vi "CLEARPATH CONTROL SYSTEM 1 AXIS.vi"() -> ()   [LabVIEW 2014]
uses:
  Control 1.ctl
  54e35cf9-3849-4311-9828-ef4f6905ae2a.vi
  83293444-dc6f-4323-ab08-cbfa26563ffd.vi
  <vilib>/Instr/_visa.llb/VISA Flush IO Buffer Mask.ctl
  b9a6dcee-82f6-4e18-8d36-9c0f5dd18835.vi
  <vilib>/Instr/_visa.llb/VISA Configure Serial Port (Instr).vi
panel:
  in  "?":bool
  in  "Y Positions (0<Y<35)":dbl[](array[numeric])
  in  "X Positions (0<X<38)":dbl[](array[numeric])
  # "End Command:\n10000"
  # "There can be no values after 10000, causes the motor to rotate infinitely. To delete a cell, \nright click on the cell, then select, Data Operations -> Delete Element. \n10000 MUST BE THE LAST COMMAND."
  # "System operates by moving to a given Y-Value,\nthen iterates through all X values. After all Y-Values\nare complete the program waits for user confirmation\nthen returns to (0,0)."
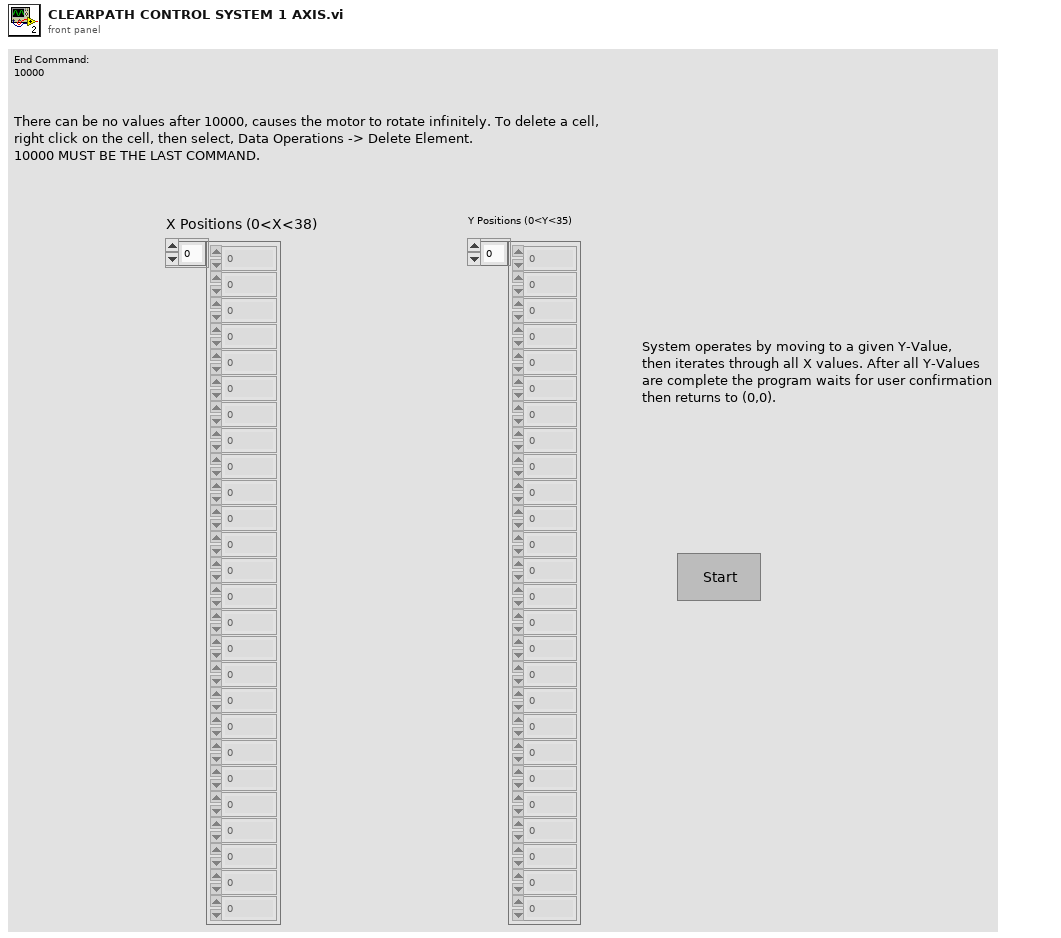
[diagram p1: front panel]
types:
  T1 = typedef "Control 1.ctl" = enum16{"Start", "Init", "Await Arduino Response", "Calculate Move", "Execute Move", "Home"}
  T2 = typedef "VISA Flush IO Buffer Mask.ctl" = u16
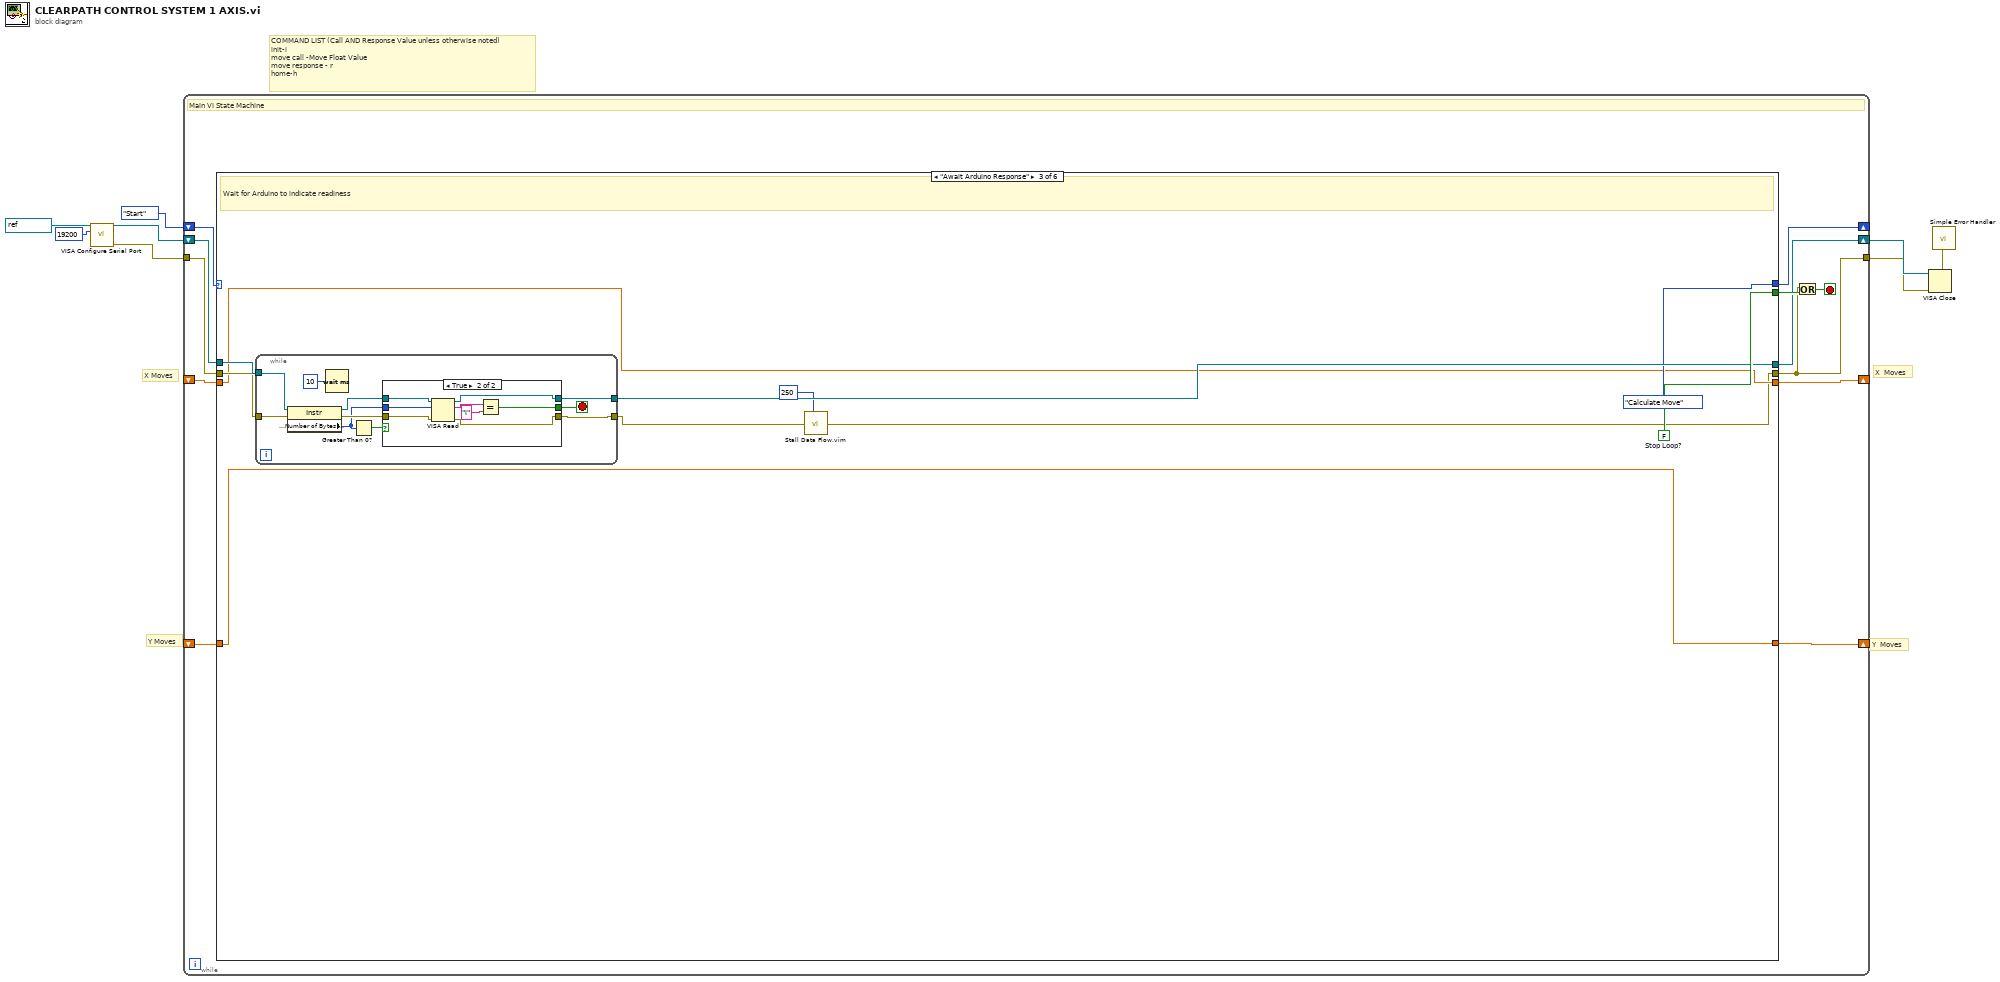
[diagram p0: block diagram]
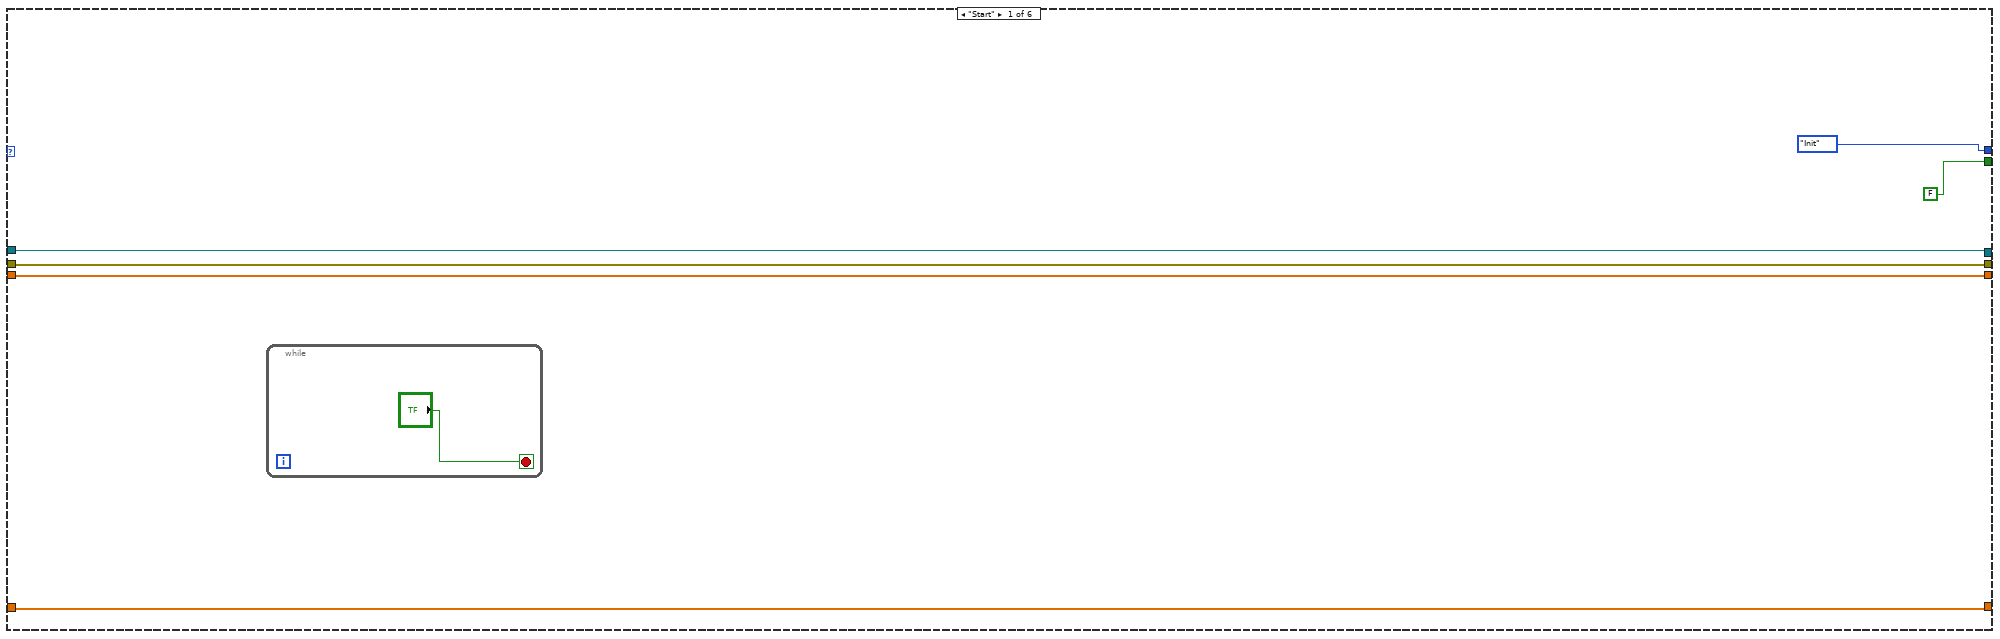
[diagram p2: hidden frame]
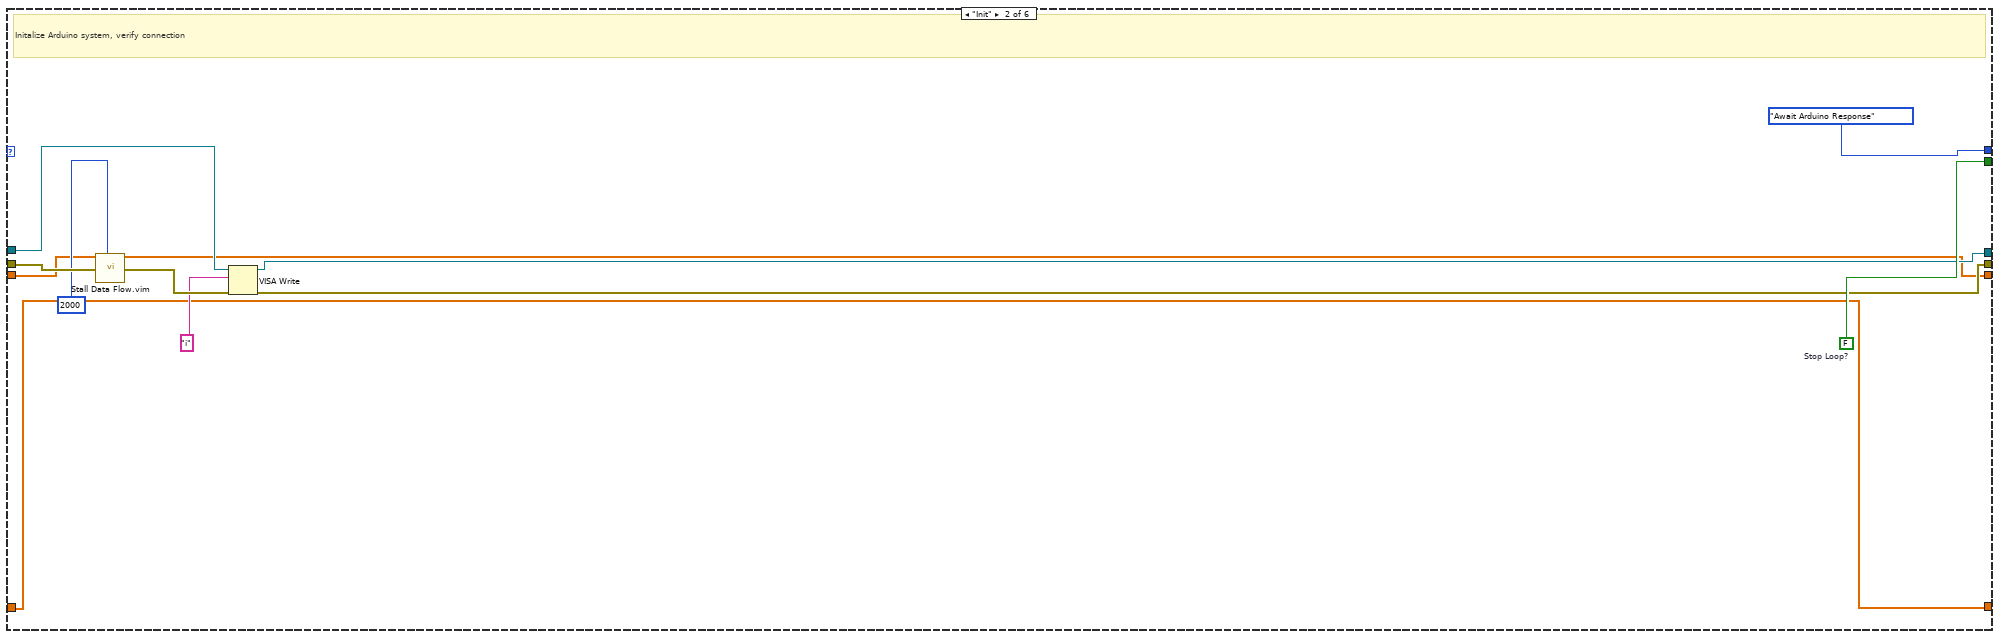
[diagram p3: hidden frame]
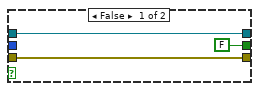
[diagram p4: hidden frame]
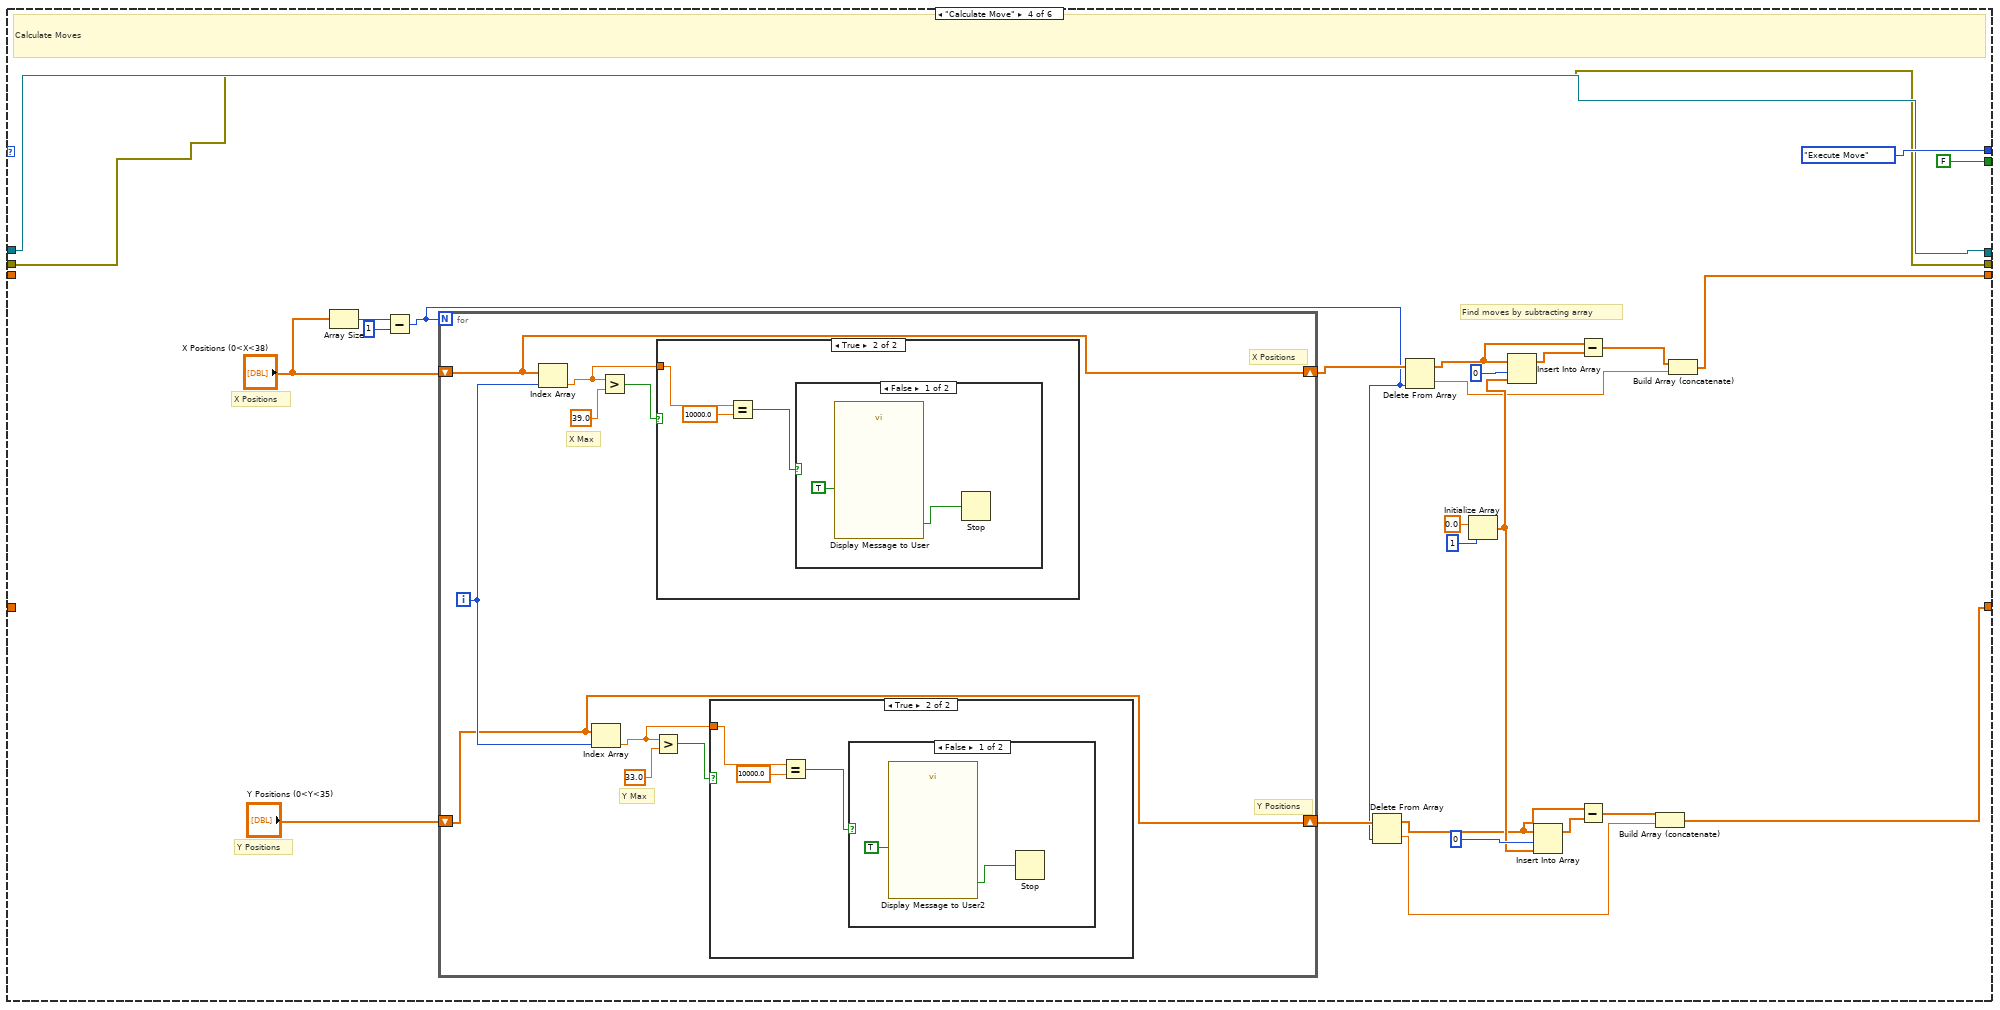
[diagram p5: hidden frame]
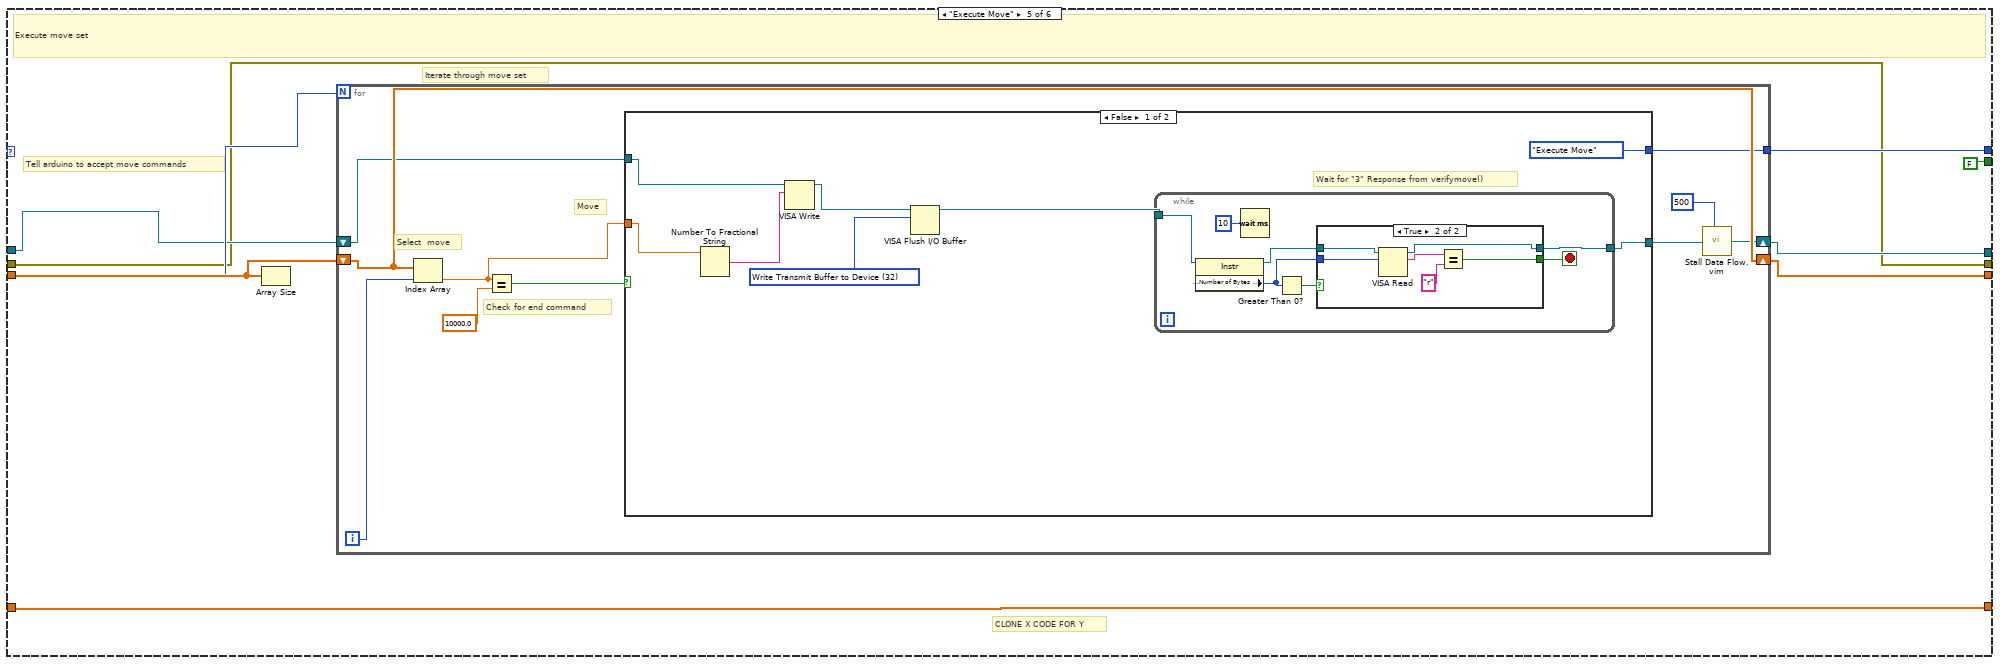
[diagram p10: hidden frame]
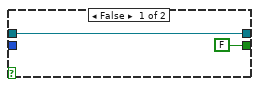
[diagram p11: hidden frame]
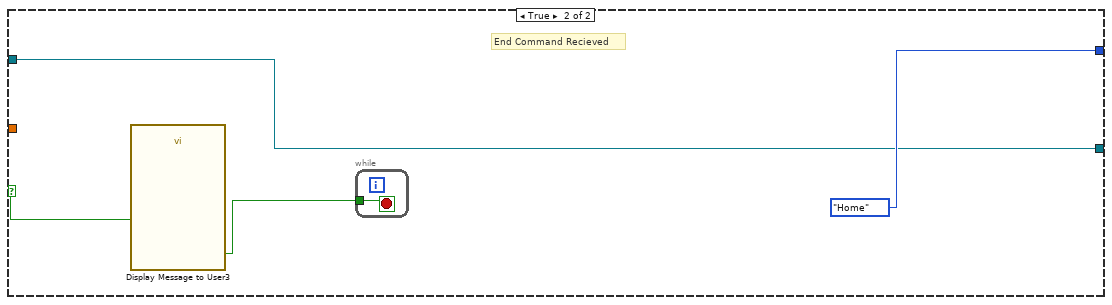
[diagram p12: hidden frame]
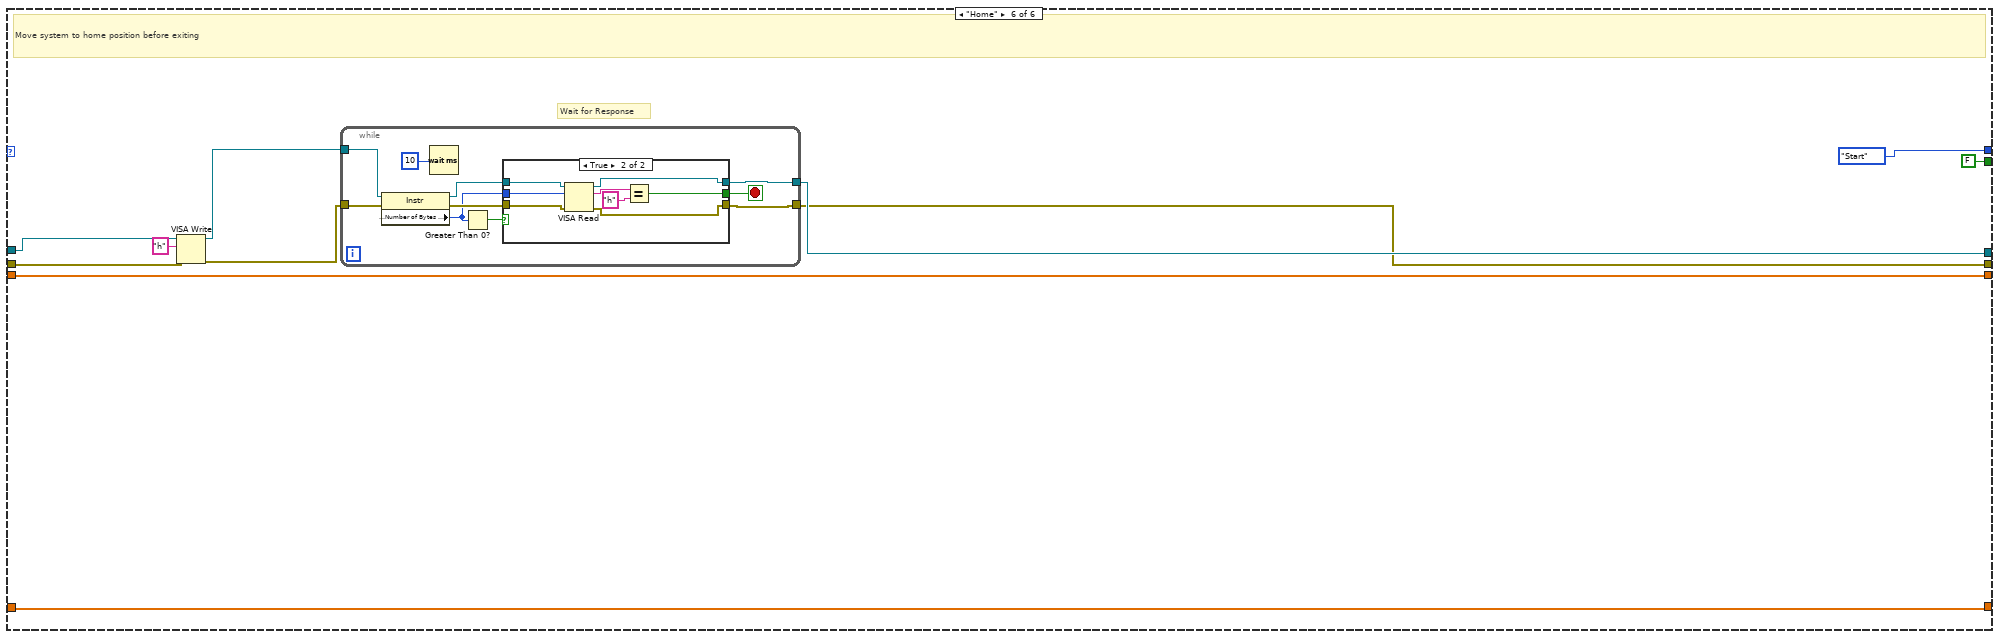
[diagram p13: hidden frame]
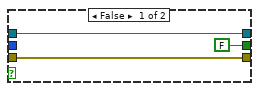
[diagram p14: hidden frame]
diagram:
  # "COMMAND LIST (Call AND Response Value unless otherwise noted)\ninit-i\nmove call -Move Float Value\nmove response - r\nhome-h"
  # "Y Moves"
  # "X Moves"
  # "Y  Moves"
  # "X  Moves"
  n1 = call-poly "VISA Configure Serial Port"("VISA resource name"=refnum<visa-resource-name> "COM8", "baud rate (9600)"=u32 19200) -> ("VISA resource name out"=w6:refnum<visa-resource-name>, "error out"=w2:errorcluster)  [unwired: 12 in]
  n2 = while {
    shift-right: [w19] -> _
    shift-left: Control_1."Start" -> [w20]
    shift-right: [w15] -> w5
    shift-left: w6 -> [w16]
    shift-right: [w14] -> _
    shift-left: _ -> [w12]
    shift-right: [w13] -> _
    shift-left: _ -> [w11]
    tunnel: w2 -> [w10]
    tunnel: [w9] -> w1
    stop <- w17 stop-if-true
    # "Main VI State Machine"
    n3 = case shown="\"Await Arduino Response\"" w20 {
      tunnel: [Control_1."Init" Control_1."Await Arduino Response" Control_1."Calculate Move" Control_1."Execute Move" w118 Control_1."Start"] -> w19
      tunnel: [FALSE w38 w48 FALSE FALSE FALSE ("Stop Loop?")] -> w18
      tunnel: w16 -> [w26 w32 w47 w93 w116 w168]
      tunnel: w10 -> [w25 w34 w46 w92 w115 w167]
      tunnel: [w26 w35 w45 w93 w117 w163] -> w15
      tunnel: [w25 w36 w40 w92 w115 w162] -> w9
      tunnel: [w24 w29 w43 w71 w120 w170] -> w14
      tunnel: [w23 w28 w42 w70 w122 w169] -> w13
      tunnel: w12 -> [w24 w29 w43 _ w121 w170]
      tunnel: w11 -> [w23 w28 w42 _ w122 w169]
      frame "Start" {
        n4 = while {
          stop <- "?" stop-if-true
        }
      }
      frame "Init" {
        w38 = FALSE  # Stop Loop?
        # "Initalize Arduino system, verify connection"
        n5 = call "Stall Data Flow.vim"("value in"=w34, "milliseconds to wait"=u32 2000) -> ("value out"=w33:errorcluster)  [unwired: 1 out]
        n6 = VISA Write(VISA resource name=w32, write buffer="i", error in (no error)=w33) -> (VISA resource name out=w35:refnum<visa-resource-name>, error out=w36:errorcluster)  [unwired: 1 out]
      }
      frame "Await Arduino Response" {
        w48 = FALSE  # Stop Loop?
        # "Wait for Arduino to indicate readiness"
        n7 = while {
          tunnel: w47 -> [w58]
          tunnel: w46 -> [w57]
          tunnel: [w51] -> w45
          tunnel: [w50] -> w41
          stop <- w52 stop-if-true
          n8 = property class="Instr"(reference=w58, error in=w57) -> (reference out=w55:refnum<visa-resource-name>, error out=w54:errorcluster, "Serial Settings:Number of Bytes at Serial Port"=w53:u32)
          n9 = Wait (ms)(milliseconds to wait=u32 10) -> ()  [unwired: 1 out]
          n10 = Greater Than 0?(x=w53) -> (x > 0?=w56:bool)
          n11 = case shown="True" w56 {
            tunnel: w55 -> [w61 w69]
            tunnel: w54 -> [w60 w68]
            tunnel: w53 -> [_ w67]
            tunnel: [FALSE w63] -> w52
            tunnel: [w61 w65] -> w51
            tunnel: [w60 w64] -> w50
            frame False {
            }
            frame True {
              n12 = VISA Read(VISA resource name=w69, byte count=w67, error in (no error)=w68) -> (VISA resource name out=w65:refnum<visa-resource-name>, read buffer=w62:string, error out=w64:errorcluster)  [unwired: 1 out]
              n13 = Equal?(x=w62, y="i") -> (x = y?=w63:bool)
            }
          }
        }
        n14 = call "Stall Data Flow.vim"("value in"=w41, "milliseconds to wait"=u32 250) -> ("value out"=w40:errorcluster)  [unwired: 1 out]
      }
      frame "Calculate Move" {
        # "Find moves by subtracting array"
        # "X Positions"
        # "Y Positions"
        # "Calculate Moves"
        n15 = Array Size(array="X Positions (0<X<38)") -> (size(s)=w87:i32)
        n16 = Subtract(x=w87, y=1) -> (x-y=w76:i32)
        n17 = for {
          N: w76 -> [_]
          shift-right: [w97] -> w89
          shift-left: "X Positions (0<X<38)" -> [w97]
          shift-right: [w96] -> w88
          shift-left: "Y Positions (0<Y<35)" -> [w96]
          i -> [w98]
          # "Y Max"
          # "X Max"
          # "Y Positions"
          # "X Positions"
          n18 = Index Array(array=w97, index=w98) -> (element=w102:dbl)
          n19 = Index Array(array=w96, index=w98) -> (element=w99:dbl)
          n20 = Greater?(x=w102, y=39.0) -> (0:w103:bool)
          n21 = Greater?(x=w99, y=33.0) -> (0:w100:bool)
          n22 = case shown="True" w103 {
            tunnel: w102 -> [_ w112]
            frame False {
            }
            frame True {
              n23 = Equal?(x=w112, y=10000.0) -> (x = y?=w110:bool)
              n24 = case shown="False" w110 {
                frame False {
                  n25 = call "Display Message to User"("Enable"=TRUE) -> ("OK"=w113:bool)  [unwired: 9 in, 1 out]
                  n26 = Stop(stop? (T)=w113) -> ()
                }
                frame True {
                }
              }
            }
          }
          n27 = case shown="True" w100 {
            tunnel: w99 -> [_ w107]
            frame False {
            }
            frame True {
              n28 = Equal?(x=w107, y=10000.0) -> (x = y?=w105:bool)
              n29 = case shown="False" w105 {
                frame False {
                  n30 = call "Display Message to User2"("Enable"=TRUE) -> ("OK"=w108:bool)  [unwired: 9 in, 1 out]
                  n31 = Stop(stop? (T)=w108) -> ()
                }
                frame True {
                }
              }
            }
          }
        }
        n32 = Delete From Array(array=w88, index=w76) -> (deleted portion=w73:dbl, array with subset deleted=w77:dbl[])  [unwired: 1 in]
        n33 = Delete From Array(array=w89, index=w76) -> (deleted portion=w72:dbl, array with subset deleted=w80:dbl[])  [unwired: 1 in]
        n34 = Initialize Array(0.0 ("element"), 1 ("dimension size")) -> (w81:dbl[])
        n35 = Insert Into Array(array=w80, index=0, new element=w81) -> (w79:dbl[])
        n36 = Insert Into Array(array=w77, index=0, new element=w81) -> (w78:dbl[])
        n37 = Subtract(x=w80, y=w79) -> (x-y=w75:dbl[])
        n38 = Subtract(x=w77, y=w78) -> (x-y=w74:dbl[])
        n39 = Build Array (concatenate)(w74, w73) -> (w70:dbl[])
        n40 = Build Array (concatenate)(w75, w72) -> (w71:dbl[])
      }
      frame "Execute Move" {
        # "Tell arduino to accept move commands"
        # "Iterate through move set"
        # "CLONE X CODE FOR Y"
        # "Execute move set"
        n41 = Array Size(array=w121) -> (size(s)=w119:i32)
        n42 = for {
          N: w119 -> [_]
          shift-right: [w129] -> w120
          shift-left: w121 -> [w129]
          tunnel: [w128] -> w118
          shift-right: [w125] -> w117
          shift-left: w116 -> [w127]
          i -> [w133]
          # "Check for end command"
          # "Move"
          # "Select  move"
          n43 = Index Array(array=w129, index=w133) -> (element=w130:dbl)
          n44 = Equal?(x=w130, y=10000.0) -> (x = y?=w131:bool)
          n45 = case shown="False" w131 {
            selector: w131 -> [_ w159]
            tunnel: w130 -> [w138 _]
            tunnel: [Control_1."Execute Move" Control_1."Home"] -> w128
            tunnel: w127 -> [w139 w157]
            tunnel: [w140 w157] -> w126
            frame False {
              w134 = T2 32 items=["Flush Receive Buffer"=16, "Write Transmit Buffer to Device"=32, "Flush Receive Buffer (No I/O)"=64, "Flush Transmit Buffer"=128] ("Mask")
              # "Wait for \"3\" Response from verifymove()"
              n46 = Number To Fractional String(number=w138) -> (F-format string=w137:string)  [unwired: 3 in]
              n47 = VISA Write(VISA resource name=w139, write buffer=w137) -> (VISA resource name out=w136:refnum<visa-resource-name>)  [unwired: 1 in, 2 out]
              n48 = VISA Flush I/O Buffer(VISA resource name=w136, mask (16)=w134) -> (VISA resource name out=w135:refnum<visa-resource-name>)  [unwired: 1 in, 1 out]
              n49 = while {
                tunnel: w135 -> [w148]
                tunnel: [w143] -> w140
                stop <- w144 stop-if-true
                n50 = property class="Instr"(reference=w148) -> (reference out=w146:refnum<visa-resource-name>, "Serial Settings:Number of Bytes at Serial Port"=w145:u32)  [unwired: 1 in, 1 out]
                n51 = Wait (ms)(milliseconds to wait=u32 10) -> ()  [unwired: 1 out]
                n52 = Greater Than 0?(x=w145) -> (x > 0?=w147:bool)
                n53 = case shown="True" w147 {
                  tunnel: w146 -> [w150 w156]
                  tunnel: w145 -> [_ w155]
                  tunnel: [FALSE w153] -> w144
                  tunnel: [w150 w154] -> w143
                  frame False {
                  }
                  frame True {
                    n54 = VISA Read(VISA resource name=w156, byte count=w155) -> (VISA resource name out=w154:refnum<visa-resource-name>, read buffer=w152:string)  [unwired: 1 in, 2 out]
                    n55 = Equal?(x=w152, y="r") -> (x = y?=w153:bool)
                  }
                }
              }
            }
            frame True {
              # "End Command Recieved"
              n56 = call "Display Message to User3"("Enable"=w159) -> ("Return to Home"=w160:bool)  [unwired: 9 in, 1 out]
              n57 = while {
                tunnel: w160 -> [w161]
                stop <- w161 stop-if-true
              }
            }
          }
          n58 = call "Stall Data Flow.vim"("value in"=w126, "milliseconds to wait"=u32 500) -> ("value out"=w125:refnum<visa-resource-name>)  [unwired: 1 out]
        }
      }
      frame "Home" {
        # "Wait for Response"
        # "Move system to home position before exiting"
        n59 = VISA Write(VISA resource name=w168, write buffer="h", error in (no error)=w167) -> (VISA resource name out=w165:refnum<visa-resource-name>, error out=w164:errorcluster)  [unwired: 1 out]
        n60 = while {
          tunnel: w165 -> [w182]
          tunnel: w164 -> [w181]
          tunnel: [w175] -> w163
          tunnel: [w174] -> w162
          stop <- w176 stop-if-true
          n61 = property class="Instr"(reference=w182, error in=w181) -> (reference out=w179:refnum<visa-resource-name>, error out=w178:errorcluster, "Serial Settings:Number of Bytes at Serial Port"=w177:u32)
          n62 = Wait (ms)(milliseconds to wait=u32 10) -> ()  [unwired: 1 out]
          n63 = Greater Than 0?(x=w177) -> (x > 0?=w180:bool)
          n64 = case shown="True" w180 {
            tunnel: w179 -> [w185 w193]
            tunnel: w178 -> [w184 w192]
            tunnel: w177 -> [_ w191]
            tunnel: [FALSE w187] -> w176
            tunnel: [w185 w189] -> w175
            tunnel: [w184 w188] -> w174
            frame False {
            }
            frame True {
              n65 = VISA Read(VISA resource name=w193, byte count=w191, error in (no error)=w192) -> (VISA resource name out=w189:refnum<visa-resource-name>, read buffer=w186:string, error out=w188:errorcluster)  [unwired: 1 out]
              n66 = Equal?(x=w186, y="h") -> (x = y?=w187:bool)
            }
          }
        }
      }
    }
    n67 = Or(x=w9, y=w18) -> (x .or. y?=w17:bool)
  }
  n68 = VISA Close(VISA resource name=w5, error in (no error)=w1) -> (error out=w7:errorcluster)
  n69 = call <vilib>:"Simple Error Handler.vi"("error in (no error)"=w7) -> ()  [unwired: 4 in, 5 out]
